vi "10K阻抗管318.vi"() -> ()   [LabVIEW 2021]
uses:
  <vilib>/Utility/file.llb/Read Delimited Spreadsheet (DBL).vi
  <vilib>/imath/engines/lvmath2/RunTimeEngine/BuiltInFunctions/win_hann2/NIMS_win_hann2.vi
  <vilib>/imath/engines/lvmath2/RunTimeEngine/ErrorHandling/NIMS_Error From Error Code.vi
  <vilib>/imath/engines/lvmath2/RunTimeEngine/BuiltInFunctions/crosspsd/NIMS_crosspsd().vi
  <instcachedir>/0/NIMS_crosspsd()_05809194815340D99CE5BEA37EA1438C.lvgen/NIMS_crosspsd()_05809194815340D99CE5BEA37EA1438C_000.vi
  <vilib>/imath/engines/lvmath2/RunTimeEngine/ErrorHandling/NIMS_Create Error From Enums.vi
  <vilib>/imath/engines/lvmath2/RunTimeEngine/ArithmeticOperatorToken/NIMS_ArithmeticOperator_rightdiv(C,C).vi
  <instcachedir>/0/NIMS_ArithmeticOperator_rightdiv(C,C)_E4A7D85CB0E0454B816AE87C89BC1049.lvgen/NIMS_ArithmeticOperator_rightdiv(C,C)_E4A7D85CB0E0454B816AE87C89BC1049_000.vi
  <vilib>/imathl/engines/lvmath/Functions/Error Handling/Create Error.vi
  <vilib>/imath/engines/lvmath2/RunTimeEngine/ArithmeticOperatorToken/NIMS_ArithmeticOperator_minus.vi
  <instcachedir>/0/NIMS_ArithmeticOperator_minus_686F2F9BA8D64789BA308312BA2E7296.lvgen/NIMS_ArithmeticOperator_minus_686F2F9BA8D64789BA308312BA2E7296_000.vi
  <vilib>/imath/engines/lvmath2/RunTimeEngine/BuiltInFunctions/cos/NIMS_cos(C).vi
  <instcachedir>/0/NIMS_cos(C)_13CB105B60204B3EA2081EF6EAFDB79A.lvgen/NIMS_cos(C)_13CB105B60204B3EA2081EF6EAFDB79A_001.vi
  <vilib>/imath/engines/lvmath2/RunTimeEngine/BuiltInFunctions/sin/NIMS_sin(C).vi
  <instcachedir>/0/NIMS_sin(C)_7FD862CD78F74733A84889D4AE021370.lvgen/NIMS_sin(C)_7FD862CD78F74733A84889D4AE021370_001.vi
  <vilib>/imath/engines/lvmath2/RunTimeEngine/ArithmeticOperatorToken/NIMS_ArithmeticOperator_times.vi
  <instcachedir>/0/NIMS_ArithmeticOperator_times_4D5EB5CC26D64553A050289FD9102F59.lvgen/NIMS_ArithmeticOperator_times_4D5EB5CC26D64553A050289FD9102F59_003.vi
  <vilib>/imath/engines/lvmath2/RunTimeEngine/BuiltInFunctions/length/NIMS_length(GV).vi
  <instcachedir>/0/NIMS_length(GV)_08A3D13377FD4E4B96F5795FBF3698FA.lvgen/NIMS_length(GV)_08A3D13377FD4E4B96F5795FBF3698FA_000.vi
  <vilib>/imath/engines/lvmath2/RunTimeEngine/RangeToken/NIMS_Range.vi
  <instcachedir>/0/NIMS_Range_55C28A69746948C3BE8F3B076E0CF496.lvgen/NIMS_Range_55C28A69746948C3BE8F3B076E0CF496_001.vi
  <vilib>/imath/engines/lvmath2/RunTimeEngine/BuiltInFunctions/fft/NIMS_fft(GV).vi
  <instcachedir>/0/NIMS_fft(GV)_4C6467FC22F84E4BA42517A07EF978B0.lvgen/NIMS_fft(GV)_4C6467FC22F84E4BA42517A07EF978B0_000.vi
  <vilib>/imath/engines/lvmath2/RunTimeEngine/ArithmeticOperatorToken/NIMS_ArithmeticOperator_plus.vi
  <instcachedir>/0/NIMS_ArithmeticOperator_plus_8086907561C54B16AC97E832CC9361D4.lvgen/NIMS_ArithmeticOperator_plus_8086907561C54B16AC97E832CC9361D4_001.vi
  <vilib>/imath/engines/lvmath2/RunTimeEngine/IndexRead/NIMS V(R2).vi
  <instcachedir>/0/NIMS V(R2)_C76619605A0E4E9F8B2FA9389712AC47.lvgen/NIMS V(R2)_C76619605A0E4E9F8B2FA9389712AC47_001.vi
  <instcachedir>/0/NIMS V(R2)_C76619605A0E4E9F8B2FA9389712AC47.lvgen/NIMS V(R2)_C76619605A0E4E9F8B2FA9389712AC47_000.vi
  <vilib>/imath/engines/lvmath2/RunTimeEngine/BuiltInFunctions/abs/NIMS_abs(signed).vi
  <instcachedir>/0/NIMS_abs(signed)_C4FCB8E6058B49B797C7C8D53CA5F6EC.lvgen/NIMS_abs(signed)_C4FCB8E6058B49B797C7C8D53CA5F6EC_006.vi
  <vilib>/imath/engines/lvmath2/RunTimeEngine/BuiltInFunctions/filter_median/NIMS_filter_median(V,I32).vi
  <instcachedir>/0/NIMS_abs(signed)_C4FCB8E6058B49B797C7C8D53CA5F6EC.lvgen/NIMS_abs(signed)_C4FCB8E6058B49B797C7C8D53CA5F6EC_001.vi
  <vilib>/imath/engines/lvmath2/RunTimeEngine/BuiltInFunctions/imag/NIMS_imag(Complex).vi
  <instcachedir>/0/NIMS_imag(Complex)_3180D40D00C843A49C2B33397F857BF3.lvgen/NIMS_imag(Complex)_3180D40D00C843A49C2B33397F857BF3_002.vi
  <vilib>/imath/engines/lvmath2/RunTimeEngine/NodeEndStatement/NIMS_NodeEndStatement_Output.vi
  <instcachedir>/0/NIMS_NodeEndStatement_Output_53EC0D466D134D7ABD903AC30B43404B.lvgen/NIMS_NodeEndStatement_Output_53EC0D466D134D7ABD903AC30B43404B_005.vi
  <vilib>/imath/engines/lvmath2/RunTimeEngine/ErrorHandling/NIMS_Finalize Error.vi
  <vilib>/addons/_NISVFA/_Generation/SoundVib_Generation.lvlib
panel:
  out "历时（秒）":dbl(slide) scale=0.0..28.0 scale format="%.1f"
  in  "mic4灵敏度（V/Pa）":dbl=0.0112 format="%.4f"
  in  "待测样品面积（mm^2）":dbl=28.0 format="%.3f"
  in  "速度系数":dbl=40.0 format="%.1f"
  in  "滑动活塞距离（m）":dbl=0.04 format="%.3f"
  in  "开始测量":bool
  in  "停止频率（Hz）":dbl=20000.0 format="%#.2f"
  in  "幅值（V）":dbl=0.1 format="%.3f"
  in  "开始频率（Hz）":dbl=10.0 format="%#.2f"
  out "测试日期":string
  in  "选项卡控件":enum32{"    阻抗    ", "    速度    ", "信号采集结果"}(tab)
  out "材料":string
  out "XY图":cluster{"out_ff":dbl[], "out_absZ":dbl[]}[](graph) caption="Z/SI Acoustic Impedance"
  out "材料 2":string
  out "XY图 2":cluster{"out_ff":dbl[], "out_absV":dbl[]}[](graph) caption="V/SI Velocity"
  out "Time waveform 3":waveform(dbl)(graph)
  out "Time waveform 1":waveform(dbl)(graph)
  out "Time waveform 2":waveform(dbl)(graph)
  out "Time waveform 4":waveform(dbl)(graph)
  in  "测试材料":string
  in  "气压（kPa）":dbl=101.0 format="%.1f"
  in  "温度（°C）":dbl=22.0 format="%.1f"
  # "传递函数法测量声阻抗（10K阻抗管）"
  # "测试条件及日期"
  # "阻抗管参数"
  # "扫频激励参数"
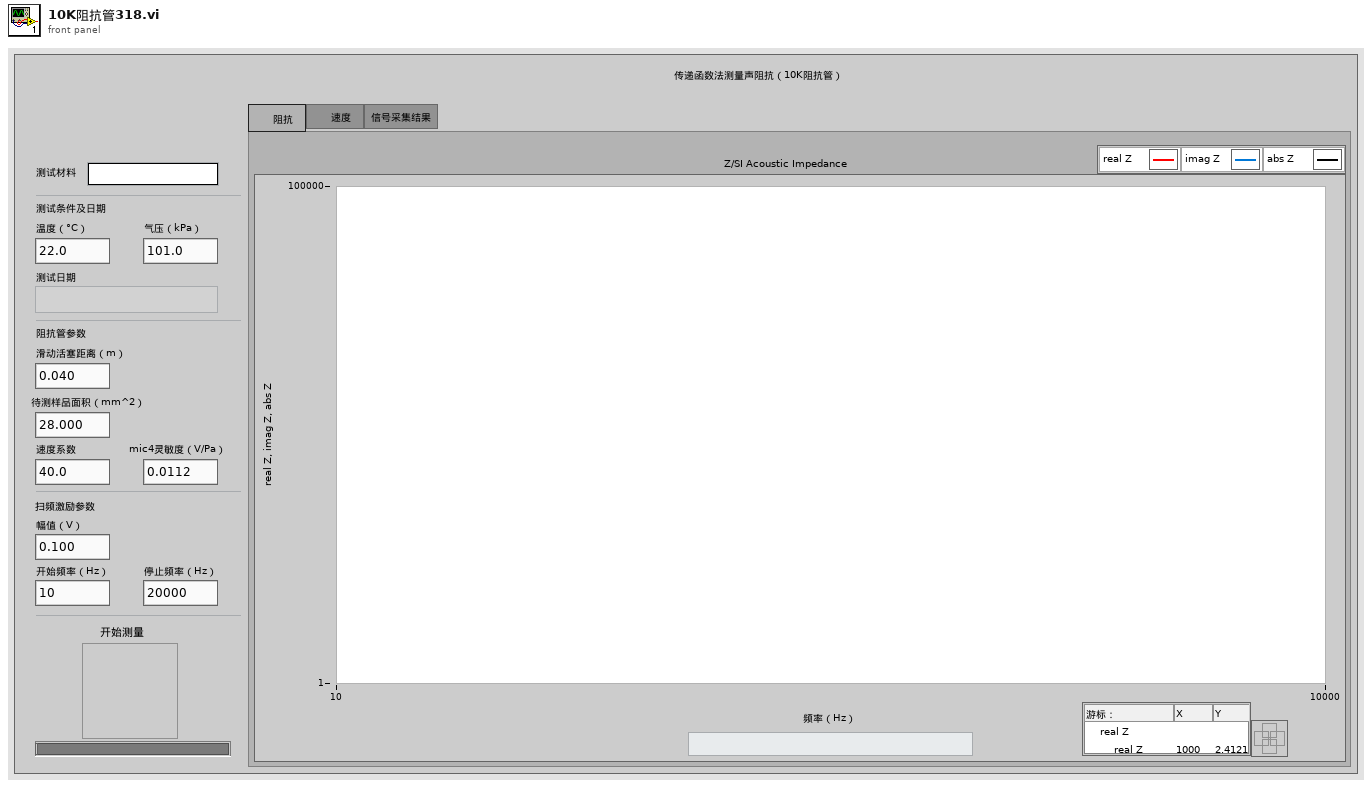
[diagram p1: front panel]
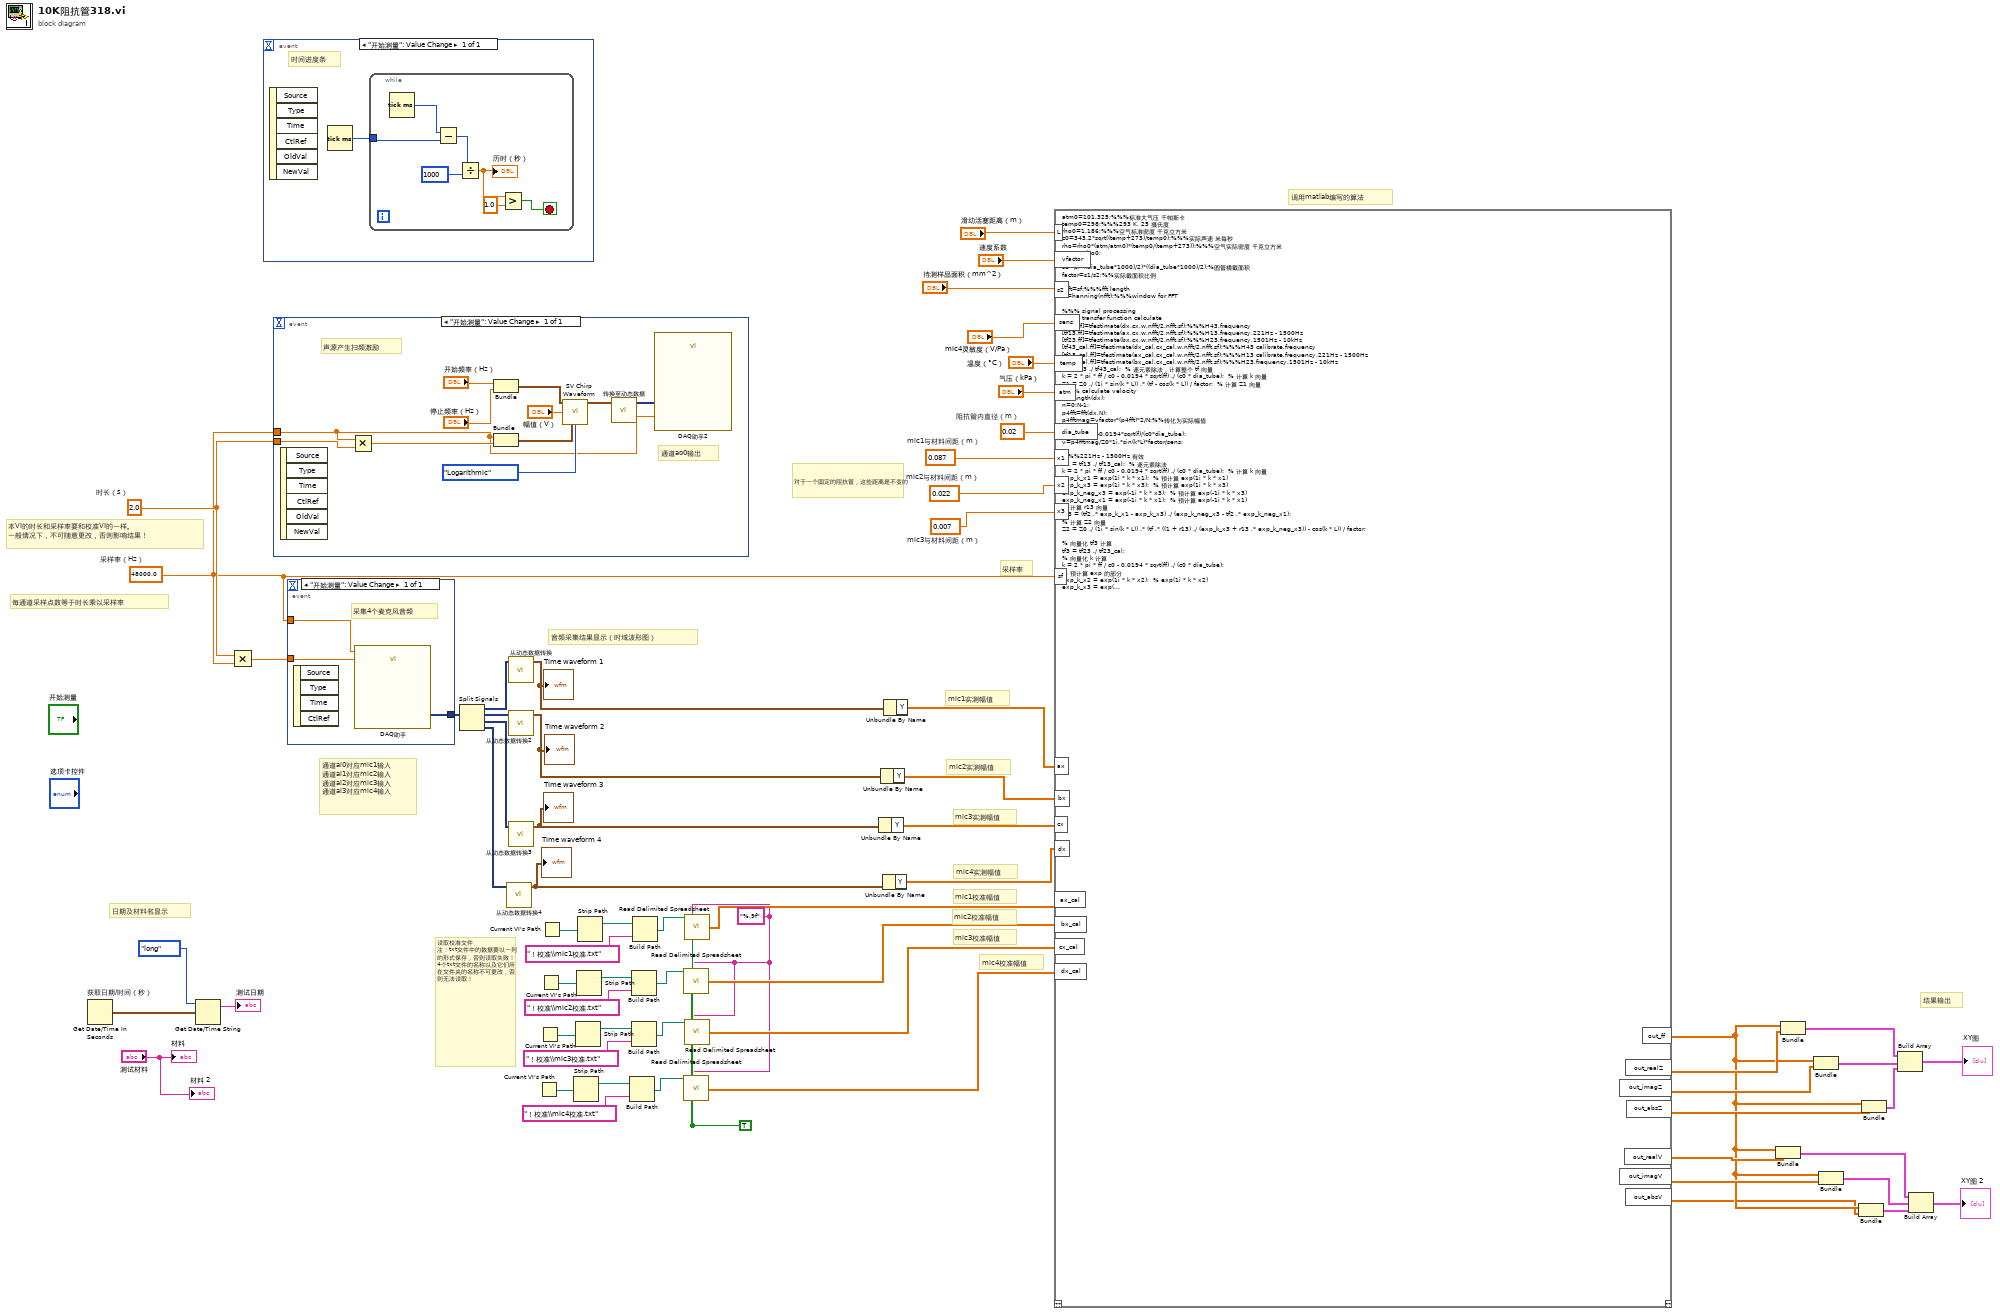
[diagram p0: block diagram]
diagram:
  w46 = 48000.0  # 采样率（Hz）
  w66 = 2.0  # 时长（s）
  w18 = 0.007  # mic3与材料间距（m）
  w47 = 0.022  # mic2与材料间距（m）
  w48 = 0.087  # mic1与材料间距（m）
  w49 = 0.02  # 阻抗管内直径（m）
  w22 = "%.9f" ("format (%.3f)")
  w50 = TRUE ("transpose? (F)")
  # "读取校准文件\n注：txt文件中的数据要以一列的形式保存，否则读取失败！ 4个txt文件的名称以及它们所在文件夹的名称不可更改，否则无法读取！"
  # "调用matlab编写的算法"
  # "每通道采样点数等于时长乘以采样率"
  # "对于一个固定的阻抗管，这些距离是不变的"
  # "采样率"
  # "本VI的时长和采样率要和校准VI的一样。\n一般情况下，不可随意更改，否则影响结果！"
  # "通道ai0对应mic1输入\n通道ai1对应mic2输入\n通道ai2对应mic3输入\n通道ai3对应mic4输入"
  # "日期及材料名显示"
  # "结果输出"
  # "mic4校准幅值"
  # "mic3校准幅值"
  # "mic2校准幅值"
  # "mic1校准幅值"
  # "mic4实测幅值"
  # "mic3实测幅值"
  # "mic2实测幅值"
  # "mic1实测幅值"
  # "音频采集结果显示（时域波形图）"
  n1 = Get Date/Time In Seconds "获取日期/时间（秒）"() -> (seconds since 1Jan1904=w62:timestamp)
  n2 = Get Date/Time String(date format (0)=enum16{"short", "long", "abbreviated"}."long" ("日期格式(0)"), seconds (now)=w62) -> (date string=→"测试日期":string)  [unwired: 1 in, 1 out]
  n3 = Multiply(x=w66, y=w46) -> (x*y=w67:dbl)
  n4 = event shown="[0] \"开始测量\": Value Change" {
    selector: _ -> [_]
    dyn-events: _ -> [_]
    timeout: _ -> [_]
    event "开始测量": Value Change {
      # "时间进度条"
      n5 = event-data() -> ()  [unwired: 1 in, 6 out]
      n6 = Tick Count (ms)() -> (millisecond timer value=w68:u32)
      n7 = while {
        tunnel: w68 -> [w74]
        stop <- w71 stop-if-true
        n8 = Tick Count (ms)() -> (millisecond timer value=w75:u32)
        n9 = Subtract(x=w75, y=w74) -> (x-y=w73:u32)
        n10 = Divide(x=w73, y=u32 1000) -> (x/y=w69:dbl)
        "历时（秒）" <- w69
        n11 = Greater?(x=w69, y=1.0) -> (0:w71:bool)
      }
    }
  }
  n12 = event shown="[0] \"开始测量\": Value Change" {
    selector: _ -> [_]
    dyn-events: _ -> [_]
    timeout: _ -> [_]
    tunnel: w66 -> [w86]
    tunnel: w46 -> [w76]
    event "开始测量": Value Change {
      # "通道ao0输出"
      # "声源产生扫频激励"
      n13 = event-data() -> ()  [unwired: 1 in, 6 out]
      n14 = Multiply(x=w76, y=w86) -> (x*y=w85:dbl)
      n15 = Bundle("开始频率（Hz）"="开始频率（Hz）", "停止频率（Hz）"="停止频率（Hz）") -> (w78:cluster{"开始频率（Hz）":dbl, "停止频率（Hz）":dbl})  [unwired: 1 in]
      n16 = Bundle("采样率（Hz）"=w76, w85) -> (w83:cluster{"采样率（Hz）":dbl, dbl})  [unwired: 1 in]
      n17 = call <vilib>:"SV Chirp Waveform.vi"("frequency range"=w78, "amplitude"="幅值（V）", "sampling info"=w83, "frequency spacing"=enum16{"Linear", "Logarithmic"}."Logarithmic") -> ("chirp signal"=w84:waveform(dbl))  [unwired: 9 in, 2 out]
      n18 = call "转换至动态数据"("Waveform"=w84) -> ("Dynamic Data Type"=w77:dynamicdata)  [unwired: 3 in]
      n19 = call "DAQ助手2"("data"=w77, "速率"=w76) -> ()  [unwired: 16 in, 2 out]
    }
  }
  n20 = event shown="[0] \"开始测量\": Value Change" {
    selector: _ -> [_]
    dyn-events: _ -> [_]
    timeout: _ -> [_]
    tunnel: [w89] -> w65
    tunnel: w46 -> [w88]
    tunnel: w67 -> [w87]
    event "开始测量": Value Change {
      # "采集4个麦克风音频"
      n21 = event-data() -> ()  [unwired: 1 in, 4 out]
      n22 = call "DAQ助手"("速率"=w88, "采样数"=w87) -> ("data"=w89:dynamicdata)  [unwired: 15 in, 2 out]
    }
  }
  n23 = Split Signals(w65) -> (w52:dynamicdata, w54:dynamicdata, w64:dynamicdata, w45:dynamicdata)  [unwired: 4 in]
  n24 = call "从动态数据转换4"("Dynamic Data Type"=w45) -> ("Waveform"=w44:waveform(dbl))  [unwired: 3 in]
  "Time waveform 4" <- w44
  n25 = call "从动态数据转换"("Dynamic Data Type"=w52) -> ("Waveform"=w60:waveform(dbl))  [unwired: 3 in]
  "Time waveform 1" <- w60
  n26 = call "从动态数据转换2"("Dynamic Data Type"=w54) -> ("Waveform"=w57:waveform(dbl))  [unwired: 3 in]
  "Time waveform 2" <- w57
  n27 = call "从动态数据转换3"("Dynamic Data Type"=w64) -> ("Waveform"=w61:waveform(dbl))  [unwired: 3 in]
  "Time waveform 3" <- w61
  n28 = Current VI's Path() -> (path=w29:path)
  n29 = Current VI's Path() -> (path=w34:path)
  n30 = Current VI's Path() -> (path=w35:path)
  n31 = Current VI's Path() -> (path=w42:path)
  n32 = Strip Path(path=w29) -> (stripped path=w30:path)  [unwired: 1 out]
  n33 = Strip Path(path=w34) -> (stripped path=w33:path)  [unwired: 1 out]
  n34 = Strip Path(path=w35) -> (stripped path=w36:path)  [unwired: 1 out]
  n35 = Strip Path(path=w42) -> (stripped path=w41:path)  [unwired: 1 out]
  n36 = Build Path(base path=w30, name or relative path="！校准\\mic4校准.txt" ("名称或相对路径")) -> (appended path=w24:path)
  n37 = Build Path(base path=w33, name or relative path="！校准\\mic3校准.txt" ("名称或相对路径")) -> (appended path=w26:path)
  n38 = Build Path(base path=w36, name or relative path="！校准\\mic2校准.txt" ("名称或相对路径")) -> (appended path=w28:path)
  n39 = Build Path(base path=w41, name or relative path="！校准\\mic1校准.txt" ("名称或相对路径")) -> (appended path=w39:path)
  n40 = call-poly <vilib>:"Read Delimited Spreadsheet.vi"("file path (dialog if empty)"=w28, "format (%.3f)"=w22, "transpose? (F)"=w50) -> ("first row"=w27:dbl[])  [unwired: 7 in, 5 out]
  n41 = call-poly <vilib>:"Read Delimited Spreadsheet.vi"("file path (dialog if empty)"=w24, "format (%.3f)"=w22, "transpose? (F)"=w50) -> ("first row"=w23:dbl[])  [unwired: 7 in, 5 out]
  n42 = call-poly <vilib>:"Read Delimited Spreadsheet.vi"("file path (dialog if empty)"=w39, "format (%.3f)"=w22, "transpose? (F)"=w50) -> ("first row"=w38:dbl[])  [unwired: 7 in, 5 out]
  n43 = call-poly <vilib>:"Read Delimited Spreadsheet.vi"("file path (dialog if empty)"=w26, "format (%.3f)"=w22, "transpose? (F)"=w50) -> ("first row"=w25:dbl[])  [unwired: 7 in, 5 out]
  n44 = Unbundle By Name(w61) -> ("Y"=w56:dbl[])
  n45 = Unbundle By Name(w57) -> ("Y"=w55:dbl[])
  n46 = Unbundle By Name(w44) -> ("Y"=w43:dbl[])
  n47 = Unbundle By Name(w60) -> ("Y"=w53:dbl[])
  n48 = mathscript code="atm0=101.325;%%%标准大气压 千帕斯卡\ntemp0=298;%%%293 K, 25 摄氏度\nrho0=1.186;%%%空气标准密度 千克立方米\nc0=343.2*sqrt((temp+273)/temp0);%%%实际声速 米每秒\nrho=rho0*(atm/atm0)*(temp0/(temp+273));%%%空气实际密度 千克立方米\nZ0=c0*rho0;\n\ns1=pi*((dia_tube*1000)/2)*((dia_tube*1000)/2);%圆管横截面积\nfactor=s1/s2;%%实际截面积比例\n\nnfft=sf;%%%fft length\nw=hanning(nfft);%%%window for FFT\n\n%%% signal processing\n%%% transfer function calculate\n[tf43,ff]=tfestimate(dx,cx,w,nfft/2,nfft,sf);%%%H43,frequency\n[tf13,ff]=tfestimate(ax,cx,w,nfft/2,nfft,sf);%%%H13,frequency,221Hz - 1500Hz\n[tf23,ff]=tfestimate(bx,cx,w,nfft/2,nfft,sf);%%%H23,frequency,1501Hz - 10kHz\n[tf43_cal,ff]=tfestimate(dx_cal,cx_cal,w,nfft/2,nfft,sf);%%%H43 calibrate,frequency\n[tf13_cal,ff]=tfestimate(ax_cal,cx_cal,w,nfft/2,nfft,sf);%%%H13 calibrate,frequency,221Hz - 1500Hz\n[tf23_cal,ff]=tfestimate(bx_cal,cx_cal,w,nfft/2,nfft,sf);%%%H23,frequency,1501Hz - 10kHz\ntf = tf43 ./ tf43_cal;  % 逐元素除法，计算整个 tf 向量\nk = 2 * pi * ff / c0 - 0.0194 * sqrt(ff) ./ (c0 * dia_tube);  % 计算 k 向量\nZ1 = Z0 ./ (1i * sin(k * L)) .* (tf - cos(k * L)) / factor;  % 计算 Z1 向量\n%%% calculate velocity\nN=length(dx);\nn=0:N-1;\np4fft=fft(dx,N);\np4fftmag=vfactor*(p4fft)*2/N;%%转化为实际幅值\nf=n*sf/N;\nk=2*pi*f/c0-0.0194*sqrt(f)/(c0*dia_tube);\nv=p4fftmag/Z0*1i.*sin(k*L)*factor/sens;\n\n%%%221Hz - 1500Hz 有效\ntf2 = tf13 ./ tf13_cal;  % 逐元素除法\nk = 2 * pi * ff / c0 - 0.0194 * sqrt(ff) ./ (c0 * dia_tube);  % 计算 k 向量\nexp_k_x1 = exp(1i * k * x1);  % 预计算 exp(1i * k * x1)\nexp_k_x3 = exp(1i * k * x3);  % 预计算 exp(1i * k * x3)\nexp_k_neg_x3 = exp(-1i * k * x3);  % 预计算 exp(-1i * k * x3)\nexp_k_neg_x1 = exp(-1i * k * x1);  % 预计算 exp(-1i * k * x1)\n% 计算 r13 向量\nr13 = (tf2 .* exp_k_x1 - exp_k_x3) ./ (exp_k_neg_x3 - tf2 .* exp_k_neg_x1);\n% 计算 Z2 向量\nZ2 = Z0 ./ (1i * sin(k * L)) .* (tf .* ((1 + r13) ./ (exp_k_x3 + r13 .* exp_k_neg_x3)) - cos(k * L)) / factor;\n\n% 向量化 tf3 计算\ntf3 = tf23 ./ tf23_cal;\n% 向量化 k 计算\nk = 2 * pi * ff / c0 - 0.0194 * sqrt(ff) ./ (c0 * dia_tube);\n% 预计算 exp 的部分\nexp_k_x2 = exp(1i * k * x2);  % exp(1i * k * x2)\nexp_k_x3 = exp(1i * k * x3);  % exp(1i * k * x3)\nexp_k_neg_x3 = exp(-1i * k * x3);  % exp(-1i * k * x3)\nexp_k_neg_x2 = exp(-1i * k * x2);  % exp(-1i * k * x2)\n% 向量化 r23 计算\nr23 = (tf3 .* exp_k_x2 - exp_k_x3) ./ (exp_k_neg_x3 - tf3 .* exp_k_neg_x2);\n% 向量化 Z3 计算\nZ3 = Z0 ./ (1i * sin(k * L)) .* (tf .* ((1 + r23) ./ (exp_k_x3 + r23 .* exp_k_neg_x3)) - cos(k * L)) / factor;\n\n %%%combine data\n% V 向量化赋值\nV = v(11:10001);\n\n% fre 和 Z 向量化赋值\nfre = [ff(11:221); ff(222:1501); ff(1502:10001)];\nZ = [Z1(11:221); Z2(222:1501); Z3(1502:10001)];\n\n%%%%data out\nout_ff=fre';\nout_absZ=(medfilt1(abs(Z),10))';\nout_realZ=(medfilt1(abs(real(Z)),10))';\nout_imagZ=(medfilt1(abs(imag(Z)),10))';\nout_absV=(medfilt1(abs(V),10))';\nout_realV=(medfilt1(abs(real(V)),10))';\nout_imagV=(medfilt1(abs(imag(V)),10))';"("ax"=w53, "bx"=w55, "cx"=w56, "ax_cal"=w38, "bx_cal"=w27, "cx_cal"=w25, "dx_cal"=w23, "temp"="温度（°C）", "atm"="气压（kPa）", "dia_tube"=w49, "x1"=w48, "x2"=w47, "sf"=w46, "dx"=w43, "L"="滑动活塞距离（m）", "vfactor"="速度系数", "s2"="待测样品面积（mm^2）", "sens"="mic4灵敏度（V/Pa）", "x3"=w18) -> ("out_ff"=w5:dbl[], "out_absZ"=w9:dbl[], "out_realZ"=w12:dbl[], "out_imagZ"=w10:dbl[], "out_absV"=w4:dbl[], "out_realV"=w7:dbl[], "out_imagV"=w6:dbl[])  [unwired: 1 in, 1 out]
  n49 = Bundle("out_ff"=w5, "out_realV"=w7) -> (w15:cluster{"out_ff":dbl[], "out_realV":dbl[]})  [unwired: 1 in]
  n50 = Bundle("out_ff"=w5, "out_realZ"=w12) -> (w11:cluster{"out_ff":dbl[], "out_realZ":dbl[]})  [unwired: 1 in]
  n51 = Bundle("out_ff"=w5, "out_imagZ"=w10) -> (w17:cluster{"out_ff":dbl[], "out_imagZ":dbl[]})  [unwired: 1 in]
  n52 = Bundle("out_ff"=w5, "out_imagV"=w6) -> (w14:cluster{"out_ff":dbl[], "out_imagV":dbl[]})  [unwired: 1 in]
  n53 = Bundle("out_ff"=w5, "out_absV"=w4) -> (w13:cluster{"out_ff":dbl[], "out_absV":dbl[]})  [unwired: 1 in]
  n54 = Bundle("out_ff"=w5, "out_absZ"=w9) -> (w16:cluster{"out_ff":dbl[], "out_absZ":dbl[]})  [unwired: 1 in]
  n55 = Build Array(w11, w17, w16) -> (→"XY图":cluster{"out_ff":dbl[], "out_absZ":dbl[]}[])
  n56 = Build Array(w15, w14, w13) -> (→"XY图 2":cluster{"out_ff":dbl[], "out_absV":dbl[]}[])
  "材料" <- "测试材料"
  "材料 2" <- "测试材料"
